vi "[SubVI]Alpha_Angle_Calculation.vi"(2 "Left Theta":dbl, 4 "Right Theta":dbl) -> (0 "Left Alpha":dbl, 1 "Right Alpha":dbl)   [LabVIEW 2019]
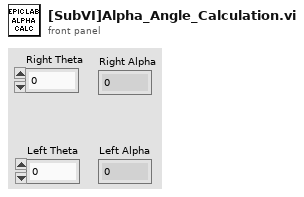
[diagram p1: front panel]
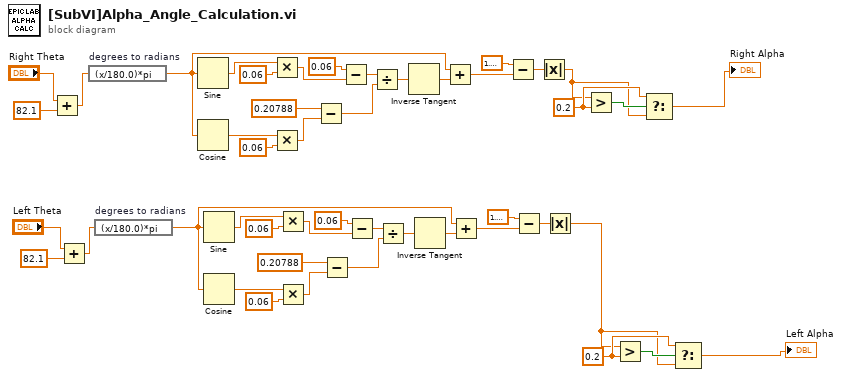
[diagram p0: block diagram]
diagram:
  w3 = 0.2 ("y")
  w7 = 0.2 ("y")
  n1 = Add(x="Right Theta", y=82.1) -> (x+y=w9:dbl)
  n2 = Add(x="Left Theta", y=82.1) -> (x+y=w12:dbl)
  n3 = expression code="(x/180.0)*pi" "degrees to radians"(w9) -> (w34:dbl)
  n4 = expression code="(x/180.0)*pi" "degrees to radians"(w12) -> (w18:dbl)
  n5 = Sine(x=w34) -> (sin(x)=w44:dbl)
  n6 = Cosine(x=w34) -> (cos(x)=w42:dbl)
  n7 = Sine(x=w18) -> (sin(x)=w28:dbl)
  n8 = Cosine(x=w18) -> (cos(x)=w26:dbl)
  n9 = Multiply(x=w44, y=0.06) -> (x*y=w43:dbl)
  n10 = Multiply(x=w42, y=0.06) -> (x*y=w39:dbl)
  n11 = Multiply(x=w28, y=0.06) -> (x*y=w27:dbl)
  n12 = Multiply(x=w26, y=0.06) -> (x*y=w23:dbl)
  n13 = Subtract(x=0.20788 ("y"), y=w39) -> (x-y=w37:dbl)
  n14 = Subtract(x=0.20788 ("y"), y=w23) -> (x-y=w21:dbl)
  n15 = Subtract(x=0.06 ("y"), y=w43) -> (x-y=w38:dbl)
  n16 = Subtract(x=0.06 ("y"), y=w27) -> (x-y=w22:dbl)
  n17 = Divide(x=w38, y=w37) -> (x/y=w36:dbl)
  n18 = Divide(x=w22, y=w21) -> (x/y=w20:dbl)
  n19 = Inverse Tangent(1:w36) -> (0:w35:dbl)
  n20 = Inverse Tangent(1:w20) -> (0:w19:dbl)
  n21 = Add(x=w34, y=w35) -> (x+y=w33:dbl)
  n22 = Add(x=w18, y=w19) -> (x+y=w17:dbl)
  n23 = Subtract(x=1.5707963267948966, y=w33) -> (x-y=w31:dbl)
  n24 = Subtract(x=1.5707963267948966, y=w17) -> (x-y=w15:dbl)
  n25 = Absolute Value(x=w31) -> (abs(x)=w6:dbl)
  n26 = Absolute Value(x=w15) -> (abs(x)=w1:dbl)
  n27 = Greater?(x=w6, y=w7) -> (0:w8:bool)
  n28 = Greater?(x=w1, y=w3) -> (0:w4:bool)
  n29 = Select(t=w7, s=w8, f=w6) -> (s? t:f=→"Right Alpha":dbl)
  n30 = Select(t=w3, s=w4, f=w1) -> (s? t:f=→"Left Alpha":dbl)
